vi "Begin.vi"() -> (0 "error out":errorcluster)   [LabVIEW 2011]
doc: "Called before other user functions, this VI is expected to open initial I/O refnums, load in file data, and do all program initialization. Notice that the <B>error out</B> terminal is simply used for data flow. Wiring it to other structures or subVIs ensures that this VI runs first."
uses:
  Robot Ctl.ctl
  Robot Global Data.vi
  <vilib>/Rock Robotics/WPI/Camera/WPI_CameraWhite Balance Values.ctl
  <vilib>/Rock Robotics/WPI/Camera/WPI_CameraExposure Values.ctl
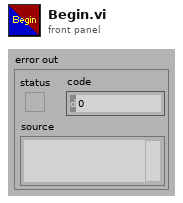
[diagram p1: front panel]
types:
  T1 = typedef "WPI_CameraExposure Values.ctl" = enum16{"Auto", "Flicker-free 50 Hz", "Flicker-free 60 Hz", "Hold current"}
  T2 = typedef "WPI_CameraWhite Balance Values.ctl" = enum16{"Auto", "Fixed indoor", "Fixed outdoor 1", "Fixed outdoor 2", "Fixed fluorescent 1", "Fixed fluorescent 2", "Hold current"}
  T3 = typedef "Robot Ctl.ctl" = enum16{"Competition", "Practice"}
  T4 = typedef "WPI_CameraImageSize.ctl" = enum16{"640x480", "320x240", "160x120"}
  T5 = typedef "WPI_CameraDevRef.ctl" = cluster{"Camera Address":string, "CameraStatus":errorcluster, "Acquire Image Notifier":refnum<notifier>}
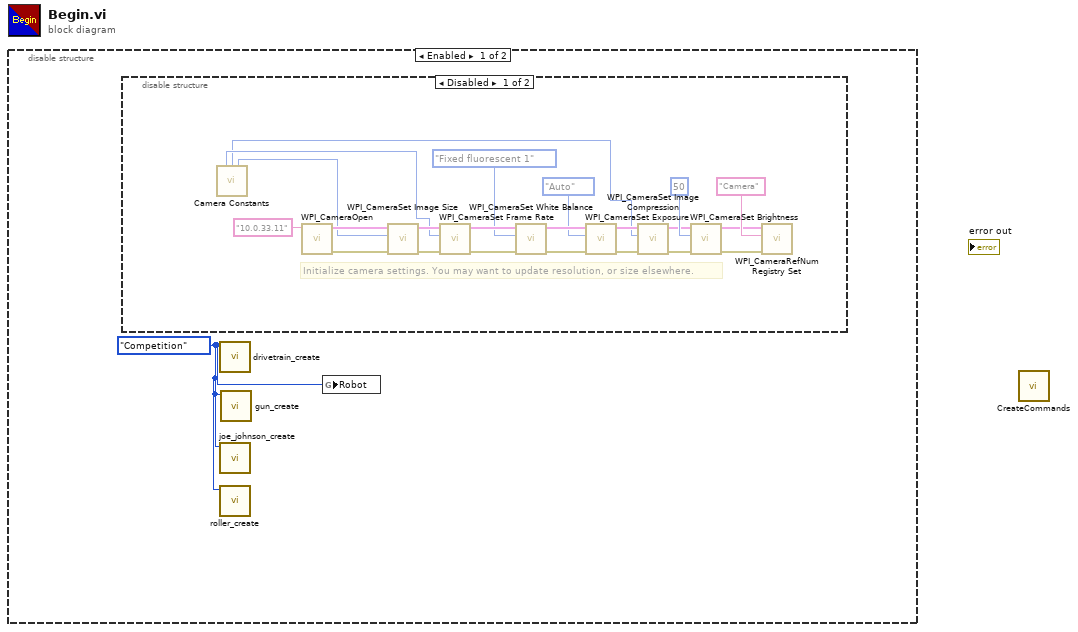
[diagram p0: block diagram]
diagram:
  n1 = disable-structure shown="Enabled" {
    frame Enabled {
      w1 = Robot_Ctl."Competition" ("Robot")
      n2 = disable-structure shown="Disabled" {
        frame Disabled {
          # "Initialize camera settings. You may want to update resolution, or size elsewhere."
          n3 = call "Camera Constants.vi"() -> ("fps robot"=w3:i32, "compression robot"=w2:i32, "img size robot"=w4:T4)  [unwired: 5 in, 8 out]
          n4 = call <vilib>:"WPI_CameraOpen.vi"("Camera Address"="10.0.33.11") -> ("error out"=w15:errorcluster, "CameraDevRef"=w16:T5)  [unwired: 1 in, 8 out]
          n5 = call <vilib>:"WPI_CameraSet Image Size.vi"("error in (no error)"=w15, "Image Size"=w4, "CameraDevRef"=w16) -> ("error out"=w14:errorcluster, "CameraDevRef Out"=w17:T5)  [unwired: 7 out]
          n6 = call <vilib>:"WPI_CameraSet Frame Rate.vi"("error in (no error)"=w14, "Frame Rate (fps)"=w3, "CameraDevRef"=w17) -> ("error out"=w13:errorcluster, "CameraDevRef Out"=w19:T5)  [unwired: 7 out]
          n7 = call <vilib>:"WPI_CameraSet White Balance.vi"("error in (no error)"=w13, "White Balance"=WPI_CameraWhite_Balance_Values."Fixed fluorescent 1", "CameraDevRef"=w19) -> ("error out"=w12:errorcluster, "CameraDevRef Out"=w18:T5)  [unwired: 7 out]
          n8 = call <vilib>:"WPI_CameraSet Exposure.vi"("error in (no error)"=w12, "Exposure"=WPI_CameraExposure_Values."Auto", "CameraDevRef"=w18) -> ("error out"=w11:errorcluster, "CameraDevRef Out"=w21:T5)  [unwired: 7 out]
          n9 = call <vilib>:"WPI_CameraSet Image Compression.vi"("error in (no error)"=w11, "Compression"=w2, "CameraDevRef"=w21) -> ("error out"=w10:errorcluster, "CameraDevRef Out"=w20:T5)  [unwired: 7 out]
          n10 = call <vilib>:"WPI_CameraSet Brightness.vi"("error in (no error)"=w10, "Brightness"=50, "CameraDevRef"=w20) -> ("error out"=w8:errorcluster, "CameraDevRef Out"=w9:T5)  [unwired: 7 out]
          n11 = call <vilib>:"WPI_CameraRefNum Registry Set.vi"("error in (no error)"=w8, "refnum name"="Camera", "CameraDevRef"=w9) -> ()  [unwired: 9 out]
        }
        frame Enabled {
        }
      }
      n12 = call "drivetrain_create.vi"("Robot"=w1) -> ()  [unwired: 11 in]
      n13 = call "joe_johnson_create.vi"("Robot"=w1) -> ()  [unwired: 11 in]
      n14 = call "roller_create.vi"("Robot"=w1) -> ()  [unwired: 11 in]
      n15 = call "gun_create.vi"("Robot"=w1) -> ()  [unwired: 11 in]
      n16 = global write "Robot Global Data.vi" "Robot"(w1) -> ()
    }
    frame Disabled {
    }
  }
  n17 = call "CreateCommands.vi"() -> ()  [unwired: 1 out]
